vi "Variant to XML - core - .vi"(6 "level":i32, 7 "Easy XML Options in":T1, 8 "error in (no error)":errorcluster, 10 "LabVIEW Data":variant) -> (0 "error out":errorcluster, 2 "XML String":string)   [LabVIEW 2011]
doc: "Generates an <B>XML String</B> from the data structure <B>LabVIEW Data</B>. You can enable \"pretty printing\" (to show the nesting of entities) by setting <B>indentation per level (0)</B> to specify the number of space characters per level. You can also specify custom <B>Type Formats</B> to overwrite the defaults.\n\nData names will have all space characters (\\s) replaced underscore (\"_\") characters.\n\nIf the first element of a cluster (parent) is a cluster (child) named \"attributes\", then child's elements are treated as attributes of parent. If this \"attributes\" cluster is present and there is one additional scalar element of parent having the same name as parent, then the scalar element's data is treated as the data of parent, rather than a child entity of parent.\n\nFor example, the following LabVIEW Data structure...\n\nmy_entity {\n attributes {\n version = \"2.0\"\n }\n my_entity = \"hello world!\"\n}\n\n...becomes...\n\n<my_entity version=\"2.0\">hello world!</my_entity>"
uses:
  Options API/Private/EasyXML Options - Data Cluster.ctl
  Options API/Private/EasyXML Options - Type Formatting Cluster.ctl
  Type Defs/Formatting Data Type -- Enum.ctl
  <userlib>/_OpenG.lib/lvdata/lvdata.llb/Type Descriptor Enumeration__ogtk.ctl
  <userlib>/_OpenG.lib/array/array.llb/Empty 1D Array (Variant)__ogtk.vi
panel:
  # "For recursion only - do not use"
  # "Copyright © 2006 James Kring, Inc. All rights reserved.\n\nAuthor: Jim Kring <jim.kring@jameskring.com>\n\nThis library is provided \"AS IS\" , WITHOUT WARRANTIES OR \nCONDITIONS OF ANY KIND, either express or implied.\n\nJames Kring, Inc. -- http://www.jameskring.com"
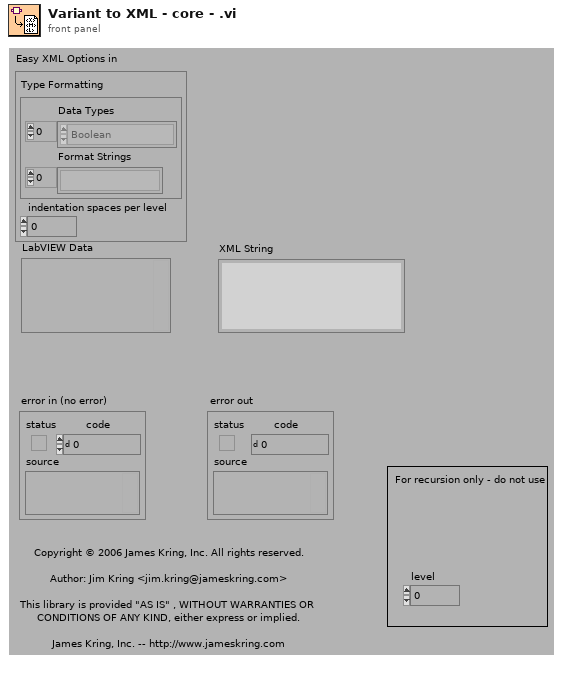
[diagram p1: front panel]
types:
  T1 = typedef "EasyXML Options - Data Cluster.ctl" = cluster{"Type Formatting":T2, "indentation spaces per level":i32}
  T2 = typedef "EasyXML Options - Type Formatting Cluster.ctl" = cluster{"Data Types":T3[], "Format Strings":string[]}
  T3 = typedef "Formatting Data Type -- Enum.ctl" = enum16{"<unknown>", "Cluster", "Array", "String", "Path", "Boolean", "Time Stamp", "Enum", "Numeric - EXT", "Numeric - DBL", "Numeric - SGL", "Numeric - I64", "Numeric - I32", "Numeric - I16", "Numeric - I8", "Numeric - U64", "Numeric - U32", "Numeric - U16", "Numeric - U8", "Numeric - CXT", "Numeric - CDB", "Numeric - CSG", "VISA Resource"}
  T4 = typedef "Type Descriptor Enumeration__ogtk.ctl" = enum8{"<Null>", "I8", "I16", "I32", "I64", "U8", "U16", "U32", "U64", "SGL", "DBL", "EXT", "CSG", "CDB", "CXT", "0x0F", "0x10", "0x11", "0x12", "0x13", "0x14", "Enum U8", "Enum U16", "Enum U32", "Enum U64", "SGL PQ", "DBL PQ", "EXT PQ", "CSG PQ", "CDB PQ", "CXT PQ", "0x1F", "0x20", "Boolean", "0x22", "0x23", "0x24", "0x25", "0x26", "0x27", "0x28", "0x29", "0x2A", "0x2B", "0x2C", "0x2D", "0x2E", "0x2F", "String", "0x31", "Path", "Pict", "0x34", "0x35", "0x36", "DAQ", "0x38", "0x39", "0x3A", "0x3B", "0x3C", "0x3D", "0x3E", "0x3F", "Array", "0x41", "0x42", "0x43", "0x44", "0x45", "0x46", "0x47", "0x48", "0x49", "0x4A", "0x4B", "0x4C", "0x4D", "0x4E", "0x4F", "Cluster", "0x51", "0x52", "Variant", "Waveform", "0x55", "0x56", "0x57", "0x58", "0x59", "0x5A", "0x5B", "0x5C", "0x5D", "0x5E", "0x5F", "0x60", "0x61", "0x62", "0x63", "0x64", "0x65", "0x66", "0x67", "0x68", "0x69", "0x6A", "0x6B", "0x6C", "0x6D", "0x6E", "0x6F", "Refnum"}
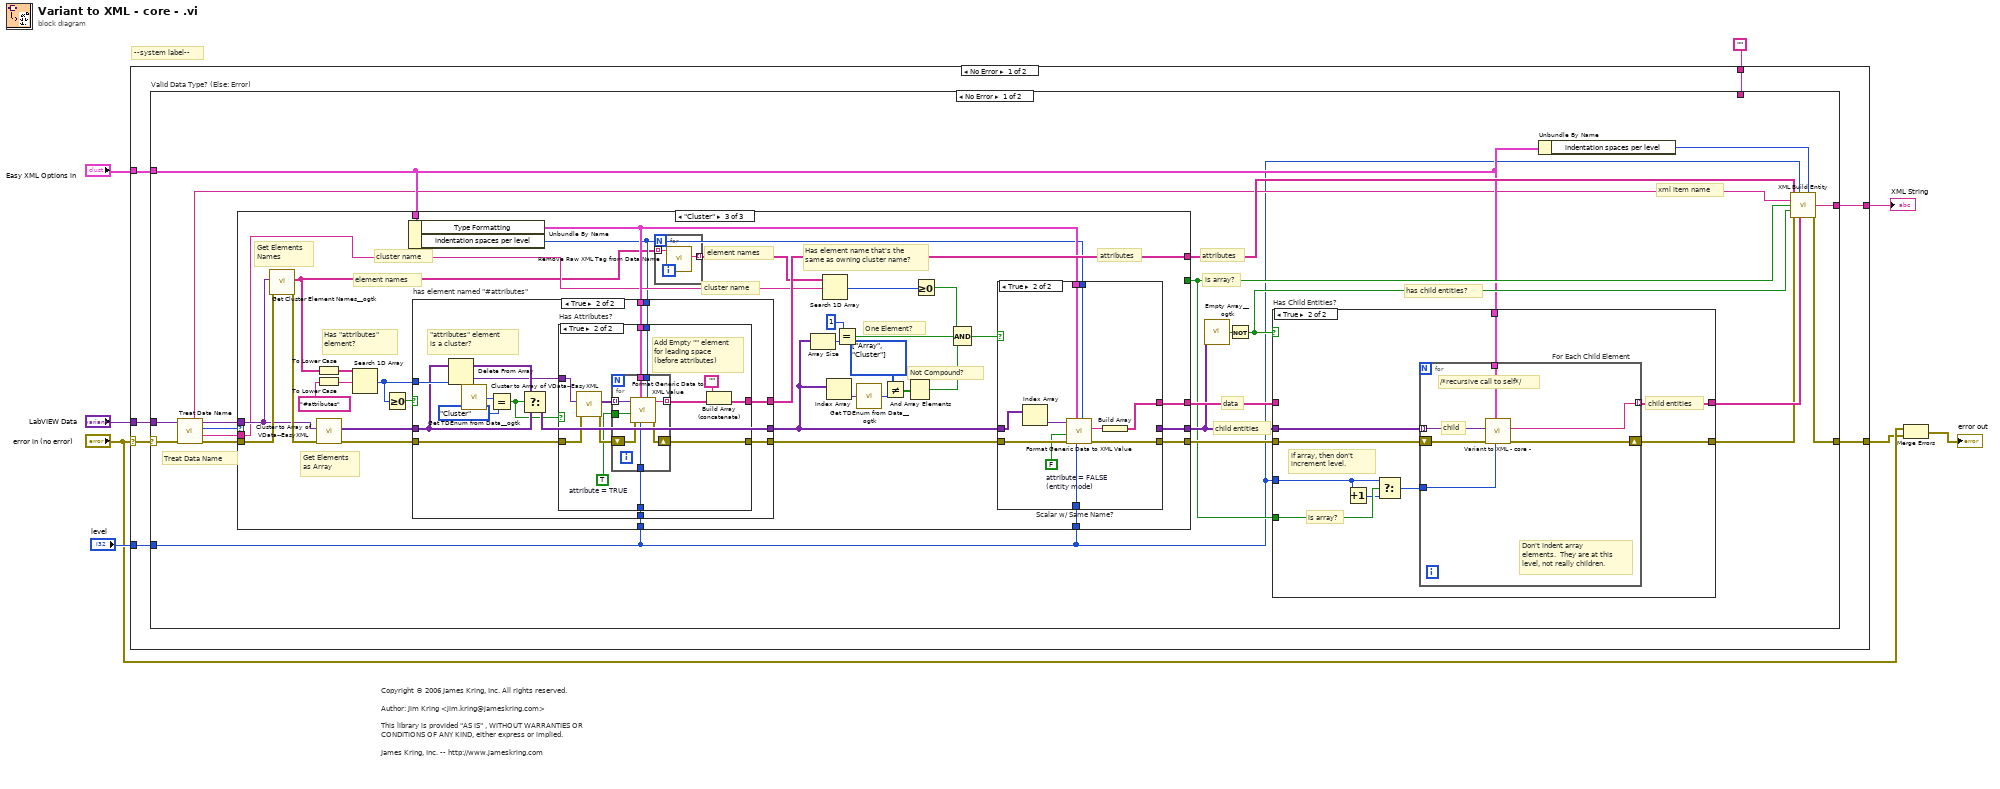
[diagram p0: block diagram]
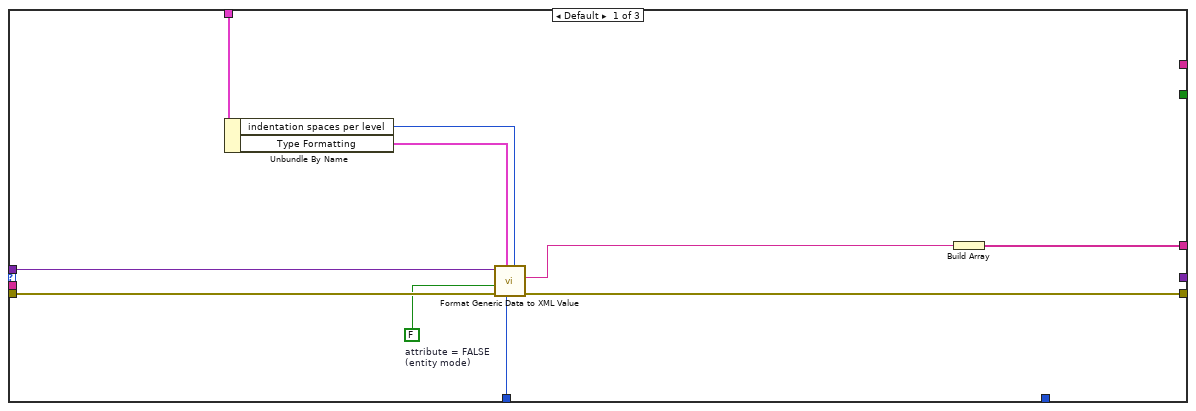
[diagram p3: hidden frame]
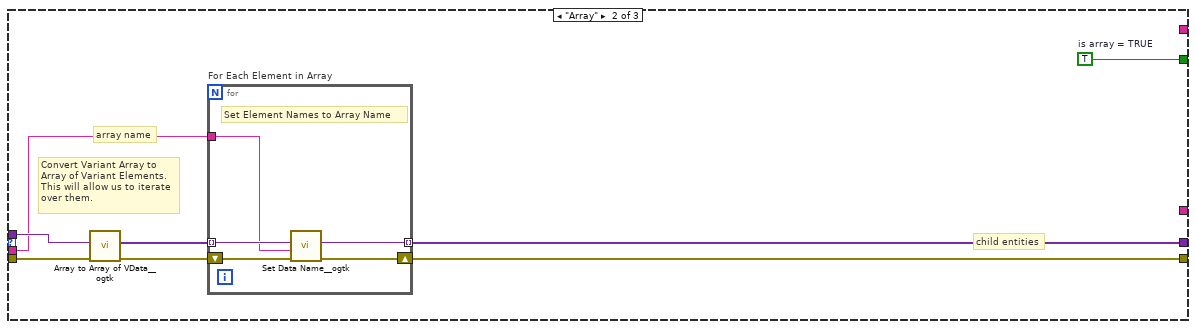
[diagram p4: hidden frame]
diagram:
  # "--system label--"
  # "Copyright © 2006 James Kring, Inc. All rights reserved.\n\nAuthor: Jim Kring <jim.kring@jameskring.com>\n\nThis library is provided \"AS IS\" , WITHOUT WARRANTIES OR \nCONDITIONS OF ANY KIND, either express or implied.\n\nJames Kring, Inc. -- http://www.jameskring.com"
  n1 = case shown="No Error" "error in (no error)" {
    selector: "error in (no error)" -> [w11 w166]
    tunnel: [w14 w166] -> w1
    tunnel: "LabVIEW Data" -> [w10 _]
    tunnel: [w15 w165] -> w7
    tunnel: "Easy XML Options in" -> [w13 _]
    tunnel: "" -> [w12 w165]
    tunnel: "level" -> [w9 _]
    frame No Error {
      n2 = case "Valid Data Type? (Else: Error)" shown="No Error" w11 {
        selector: w11 -> [w21 w163]
        tunnel: w10 -> [w20 _]
        tunnel: [w36 w164] -> w15
        tunnel: [w18 w163] -> w14
        tunnel: w13 -> [w27 _]
        tunnel: w12 -> [_ w164]
        tunnel: w9 -> [w16 _]
        frame No Error {
          # "xml item name"
          # "Treat Data Name"
          # "has child entities?"
          # "is array?"
          # "data"
          # "child entities"
          # "attributes"
          n3 = call "Treat Data Name.vi"("error in (no error)"=w21, "Data"=w20) -> ("error out"=w25:errorcluster, "untreated Data Name"=w23:string, "EasyXML Type"=w24:T3, "dup Data"=w22:variant, "treated xml name"=w19:string)  [unwired: 3 in, 2 out]
          n4 = case shown="\"Cluster\"" w24 {
            tunnel: [w58 _ w111] -> w33
            tunnel: w25 -> [w63 w70 w110]
            tunnel: [_ _ w103] -> w35
            tunnel: w27 -> [w61 _ w102]
            tunnel: [w62 w66 w101] -> w34
            tunnel: w22 -> [w60 w71 w100]
            tunnel: [_ w68 w99] -> w30
            tunnel: w23 -> [_ w65 w82]
            tunnel: [_ w64 _] -> w28
            tunnel: w16 -> [w55 _ w81]
            tunnel: w16 -> [_ _ w79]
            frame Default {
              w56 = FALSE  # attribute = FALSE (entity mode)
              n5 = Unbundle By Name(w61) -> ("indentation spaces per level"=w54:i32, "Type Formatting"=w57:T2)
              n6 = call "Format Generic Data to XML Value.vi"("spaces per level"=w54, "level"=w55, "Type Formatting"=w57, "error in (no error)"=w63, "attribute? (F: entity)"=w56, "LabVIEW Data"=w60) -> ("error out"=w62:errorcluster, "value"=w59:string)  [unwired: 2 in, 2 out]
              n7 = Build Array(w59) -> (w58:string[])
            }
            frame "Array" {
              w64 = TRUE  # is array = TRUE
              # "array name"
              # "child entities"
              # "Convert Variant Array to Array of Variant Elements.  This will allow us to iterate over them."
              n8 = call <userlib>:"Array to Array of VData__ogtk.vi"("error in (no error)"=w70, "MultiD Array"=w71) -> ("error out"=w67:errorcluster, "1D Array of Variants"=w69:variant[])  [unwired: 8 in]
              n9 = for "For Each Element in Array" {
                tunnel: w69 -> [w76] mode=indexing
                tunnel: [w75] -> w68 mode=indexing
                shift-right: [w74] -> w66
                shift-left: w67 -> [w73]
                tunnel: w65 -> [w72]
                # "Set Element Names to Array Name"
                n10 = call <userlib>:"Set Data Name__ogtk.vi"("error in (no error)"=w73, "Data Name"=w72, "Data"=w76) -> ("error out"=w74:errorcluster, "Renamed Data"=w75:variant)  [unwired: 7 in]
              }
            }
            frame "Cluster" {
              w91 = T4[] [enum."Array", enum."Cluster"] items=["<Null>", "I8", "I16", "I32", "I64", "U8", "U16", "U32", "U64", "SGL", "DBL", "EXT", "CSG", "CDB", "CXT", "0x0F", "0x10", "0x11", "0x12", "0x13", "0x14", "Enum U8", "Enum U16", "Enum U32", "Enum U64", "SGL PQ", "DBL PQ", "EXT PQ", "CSG PQ", "CDB PQ", "CXT PQ", "0x1F", "0x20", "Boolean", "0x22", "0x23", "0x24", "0x25", "0x26", "0x27", "0x28", "0x29", "0x2A", "0x2B", "0x2C", "0x2D", "0x2E", "0x2F", "String", "0x31", "Path", "Pict", "0x34", "0x35", "0x36", "DAQ", "0x38", "0x39", "0x3A", "0x3B", "0x3C", "0x3D", "0x3E", "0x3F", "Array", "0x41", "0x42", "0x43", "0x44", "0x45", "0x46", "0x47", "0x48", "0x49", "0x4A", "0x4B", "0x4C", "0x4D", "0x4E", "0x4F", "Cluster", "0x51", "0x52", "Variant", "Waveform", "0x55", "0x56", "0x57", "0x58", "0x59", "0x5A", "0x5B", "0x5C", "0x5D", "0x5E", "0x5F", "0x60", "0x61", "0x62", "0x63", "0x64", "0x65", "0x66", "0x67", "0x68", "0x69", "0x6A", "0x6B", "0x6C", "0x6D", "0x6E", "0x6F", "Refnum"]
              # "cluster name"
              # "Not Compound?"
              # "One Element?"
              # "cluster name"
              # "element names"
              # "element names"
              # "Get Elements\nNames"
              # "attributes"
              # "Has element name that's the same as owning cluster name?"
              # "Has \"attributes\" element?"
              # "Get Elements\nas Array"
              n11 = call <userlib>:"Get Cluster Element Names__ogtk.vi"("error in (no error)"=w110, "Cluster"=w100) -> ("error out"=w109:errorcluster, "Element Names"=w78:string[])  [unwired: 8 in]
              n12 = To Lower Case(string=w78) -> (all lower case string=w85:string[])
              n13 = To Lower Case(string="#attributes" ("Data Name")) -> (all lower case string=w83:string)
              n14 = call "Cluster to Array of VData--EasyXML.vi"("error in (no error)"=w109, "Cluster"=w100) -> ("error out"=w107:errorcluster, "Array of VData"=w108:variant[])  [unwired: 8 in]
              n15 = Search 1D Array(1D array=w85, element=w83) -> (index of element=w104:i32)  [unwired: 1 in]
              n16 = Greater Or Equal To 0?(x=w104) -> (x >= 0?=w105:bool)
              n17 = Unbundle By Name(w102) -> ("Type Formatting"=w97:T2, "indentation spaces per level"=w80:i32)
              n18 = case "has element named \"#attributes\"" shown="True" w105 {
                tunnel: w108 -> [w127 w138]
                tunnel: [w127 w136] -> w88
                tunnel: [w126 w134] -> w106
                tunnel: w107 -> [w126 w135]
                tunnel: w104 -> [_ w141]
                tunnel: w97 -> [_ w133]
                tunnel: [_ w131] -> w103
                tunnel: w81 -> [_ w129]
                tunnel: w80 -> [_ w128]
                frame False {
                }
                frame True {
                  # "\"attributes\" element is a cluster?"
                  n19 = Delete From Array(array=w138, index=w141) -> (deleted portion=w132:variant, array with subset deleted=w137:variant[])  [unwired: 1 in]
                  n20 = call <userlib>:"Get TDEnum from Data__ogtk.vi"("Data"=w132) -> ("Type Descriptor Enumeration"=w140:T4)  [unwired: 4 in]
                  n21 = Equal?(x=w140, y=Type_Descriptor_Enumeration__ogtk."Cluster" ("Type Descriptor Enumeration")) -> (x = y?=w130:bool)
                  n22 = Select(t=w137, s=w130, f=w138) -> (s? t:f=w136:variant[])
                  n23 = case "Has Attributes?" shown="True" w130 {
                    tunnel: w135 -> [w142 w152]
                    tunnel: [w142 w151] -> w134
                    tunnel: w133 -> [_ w150]
                    tunnel: w132 -> [_ w149]
                    tunnel: [_ w147] -> w131
                    tunnel: w129 -> [_ w144]
                    tunnel: w128 -> [_ w143]
                    frame False {
                    }
                    frame True {
                      w145 = TRUE  # attribute = TRUE
                      # "Add Empty \"\" element for leading space (before attributes)"
                      n24 = call "Cluster to Array of VData--EasyXML.vi"("error in (no error)"=w152, "Cluster"=w149) -> ("error out"=w154:errorcluster, "Array of VData"=w153:variant[])  [unwired: 8 in]
                      n25 = for {
                        tunnel: w150 -> [w162]
                        tunnel: w153 -> [w159] mode=indexing
                        tunnel: [w158] -> w146 mode=indexing
                        shift-right: [w160] -> w151
                        shift-left: w154 -> [w161]
                        tunnel: w145 -> [w157]
                        tunnel: w144 -> [w156]
                        tunnel: w143 -> [w155]
                        n26 = call "Format Generic Data to XML Value.vi"("spaces per level"=w155, "level"=w156, "Type Formatting"=w162, "error in (no error)"=w161, "attribute? (F: entity)"=w157, "LabVIEW Data"=w159) -> ("error out"=w160:errorcluster, "Data Elements"=w158:string)  [unwired: 2 in, 2 out]
                      }
                      n27 = Build Array (concatenate)("", w146) -> (w147:string[])
                    }
                  }
                }
              }
              n28 = for {
                tunnel: w78 -> [w113] mode=indexing
                tunnel: [w112] -> w77 mode=indexing
                n29 = call "Remove Raw XML Tag from Data Name.vi"("Data Name"=w113) -> ("Data Name without #xml"=w112:string)  [unwired: 9 in, 1 out]
              }
              n30 = Array Size(array=w88) -> (size(s)=w96:i32)
              n31 = Search 1D Array(1D array=w77, element=w82) -> (index of element=w98:i32)  [unwired: 1 in]
              n32 = Index Array(array=w88) -> (element=w93:variant)  [unwired: 1 in]
              n33 = Equal?(x=1, y=w96) -> (x = y?=w94:bool)
              n34 = call <userlib>:"Get TDEnum from Data__ogtk.vi"("Data"=w93) -> ("Type Descriptor Enumeration"=w92:T4)  [unwired: 4 in]
              n35 = Not Equal?(x=w91, y=w92) -> (x != y?=w90:bool[])
              n36 = And Array Elements(Boolean array=w90) -> (logical AND=w89:bool)
              n37 = Greater Or Equal To 0?(x=w98) -> (x >= 0?=w87:bool)
              n38 = Compound Arithmetic op=AND(w87, w94, w89) -> (w86:bool)
              n39 = case "Scalar w/ Same Name?" shown="True" w86 {
                tunnel: [w115 w123] -> w101
                tunnel: [_ w122] -> w111
                tunnel: w106 -> [w115 w124]
                tunnel: w88 -> [w114 w120]
                tunnel: w97 -> [_ w125]
                tunnel: [w114 _] -> w99
                tunnel: w80 -> [_ w117]
                tunnel: w79 -> [_ w116]
                frame False {
                }
                frame True {
                  w118 = FALSE  # attribute = FALSE (entity mode)
                  n40 = Index Array(array=w120) -> (element=w119:variant)  [unwired: 1 in]
                  n41 = call "Format Generic Data to XML Value.vi"("spaces per level"=w117, "level"=w116, "Type Formatting"=w125, "error in (no error)"=w124, "attribute? (F: entity)"=w118, "LabVIEW Data"=w119) -> ("error out"=w123:errorcluster, "value"=w121:string)  [unwired: 2 in, 2 out]
                  n42 = Build Array(w121) -> (w122:string[])
                }
              }
            }
          }
          n43 = call-poly <userlib>:"Empty Array__ogtk.vi"("Array"=w30) -> ("Empty Array?"=w29:bool)  [unwired: 8 in]
          n44 = Not(x=w29) -> (.not. x?=w31:bool)
          n45 = case "Has Child Entities?" shown="True" w31 {
            tunnel: w30 -> [_ w46]
            tunnel: [w37 w40] -> w17
            tunnel: w34 -> [w37 w39]
            tunnel: w33 -> [w38 _]
            tunnel: [w38 w47] -> w32
            tunnel: w27 -> [_ w45]
            tunnel: w28 -> [_ w44]
            tunnel: w16 -> [_ w43]
            frame False {
              # "data"
            }
            frame True {
              # "is array?"
              # "child entities"
              # "if array, then don't increment level."
              n46 = Increment(x=w43) -> (x+1=w42:i32)
              n47 = Select(t=w43, s=w44, f=w42) -> (s? t:f=w41:i32)
              n48 = for "For Each Child Element" {
                shift-right: [w51] -> w40
                shift-left: w39 -> [w52]
                tunnel: w46 -> [w53] mode=indexing
                tunnel: [w50] -> w47 mode=indexing
                tunnel: w45 -> [w48]
                tunnel: w41 -> [w49]
                # "Don't indent array elements.  They are at this level, not really children."
                # "child"
                # "/*recursive call to self*/"
                n49 = call "Variant to XML - core - .vi"("level"=w49, "Easy XML Options in"=w48, "error in (no error)"=w52, "LabVIEW Data"=w53) -> ("error out"=w51:errorcluster, "XML String"=w50:string)  [unwired: 6 in]
              }
            }
          }
          n50 = Unbundle By Name(w27) -> ("indentation spaces per level"=w26:i32)
          n51 = call "XML Build Entity.vi"("Attributes"=w35, "level"=w16, "spaces per level"=w26, "Entity Name"=w19, "Is Array?"=w28, "Has Children"=w31, "error in (no error)"=w17, "Child Entities"=w32) -> ("Entity XML"=w36:string, "error out"=w18:errorcluster)  [unwired: 6 in]
        }
        frame Error {
        }
      }
    }
    frame Error {
    }
  }
  "XML String" <- w7
  n52 = Merge Errors("error in (no error)", w1) -> (→"error out":errorcluster)
